vi "StepClock.vi"(8 "error in (no error)":errorcluster, 9 "SequenceNumber":u32, 10 "address":u32, 11 "connection ID":refnum<k16>) -> (0 "error out":errorcluster, 1 "SequenceNumber out":i32, 2 "address out":u32, 3 "connection ID out":refnum<k16>)   [LabVIEW 2009]
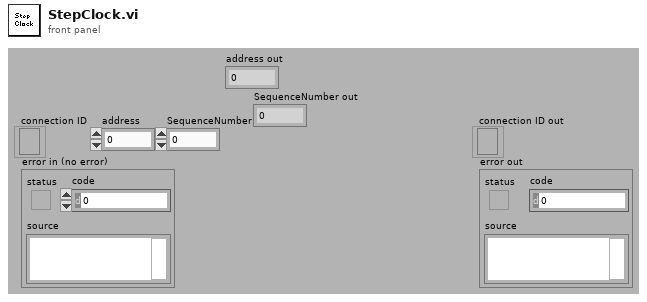
[diagram p1: front panel]
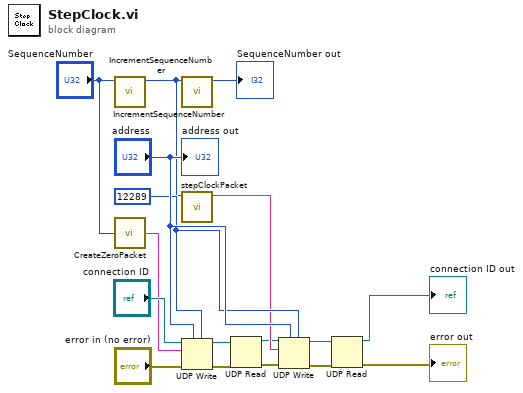
[diagram p0: block diagram]
diagram:
  w12 = u16 12289 ("port or service name")
  n1 = call "IncrementSequenceNumber.vi"("In"="SequenceNumber") -> ("Out"=w10:i32)  [unwired: 10 in]
  n2 = call "CreateZeroPacket.vi"("SequenceNumber"="SequenceNumber") -> ("ZeroPacket"=w14:string)
  n3 = call "IncrementSequenceNumber.vi"("In"=w10) -> ("Out"=→"SequenceNumber out":i32)  [unwired: 10 in]
  n4 = call "stepClockPacket.vi"("SequenceNumber"=w10) -> ("StepClockPacket"=w11:string)  [unwired: 10 in]
  n5 = UDP Write(address="address", port or service name=w12, connection ID="connection ID", data in=w14, 8:"error in (no error)") -> (error out=w7:errorcluster, 3:w8:refnum<k16>)  [unwired: 1 in]
  n6 = UDP Read(connection ID=w8, 8:w7) -> (error out=w6:errorcluster, 3:w5:refnum<k16>)  [unwired: 2 in, 3 out]
  n7 = UDP Write(address="address", port or service name=w12, connection ID=w5, data in=w11, 8:w6) -> (error out=w3:errorcluster, 3:w4:refnum<k16>)  [unwired: 1 in]
  n8 = UDP Read(connection ID=w4, 8:w3) -> (error out=→"error out":errorcluster, 3:→"connection ID out":refnum<k16>)  [unwired: 2 in, 3 out]
  "address out" <- "address"
